vi "p6.2.vi"() -> ()   [LabVIEW 2020]
panel:
  in  "Kw":dbl=2.0
  in  "N FFT dBV":i32=4096
  out "FFT dBV":dbl[](graph)
  in  "N FFT":i32=1024
  out "FFT":dbl[](graph)=[1.1102230246251565e-16, 0.1179404859776075, 0.41931414977318965, 0.7678697584481545, 0.9999999999999988, 0.9969135645094994, 0.7439410887048731, 0.34832600660220614, 4.3813988651205395e-16, -0.11515526215938783, 0.08700222996580775, 0.5306405355054225, 0.9999999999999997, 1.2397845389517068, 1.0922522743307335, 0.5984660918442707, 5.761955295844675e-16, -0.3743504024510719, -0.28699300761890545, 0.26039872656253404, 0.9999999999999997, 1.5233277475171119, 1.5039874509749693, 0.8979000853754242, 9.418075112973702e-16, -0.6926899491581942, -0.7523921491322665, -0.08040357528638686, 0.9999999999999998, 1.8908459734075165, 2.0452675115378183, 1.297288147417813, 9.08683004564401e-16, -1.1302804118304979, -1.4022740708363133, -0.5640918868488319, 1.0000000000000009, 2.430632585174213, 2.8548321612466925, 1.9060608537435746, 8.633112624768329e-16, -1.8249724926294415, -2.4568882184753864, -1.3674473641410647, 0.9999999999999997, 3.373989764053941, 4.310015993746622, 3.033921208946577, 3.612083235008795e-16, -3.2028711087728787, -4.6315288740934175, -3.0963415349348566, 0.9999999999999983, 5.6186233099847, 7.986040899784292, 6.084571725761597, 1.1893112847244443e-17, -7.629629162693573, -12.443245049139438, -10.223584372481056, 0.9999999999999952, 19.621619548856494, 40.628968402289644, 57.33600236327664, 64.0, 58.189610616642796, 41.83638559111921, 20.475666946026298, 1.0000000000000062, -11.07851134787117, -13.653150976397987, -8.485878741428298, -6.022881901310196e-16, 6.942590842860555, 9.200953695486772, 6.478864158519104, 1.0000000000000013, -3.959262953429805, -5.854026322970516, -4.068940018683909, -6.904390630761646e-16, 3.903614113749591, 5.542767590086527, 4.2477943223758015, 1.0000000000000004, -2.245864050443687, -3.702690034497498, -2.7085163602699627, -5.049791833514398e-16, 2.795263416798454, 4.1166457149068005, 3.3260438372759777, 1.0000000000000013, -1.4662824774882115, -2.683270621160191, -2.039844003183214, -2.170775191704935e-16, 2.214843977835635, 3.3488795541278797, 2.8170416573555173, 1.0, -1.015918173819969, -2.0823743678223012, -1.638237350146765, -2.802329447010364e-16, 1.8542327387573896, 2.8644900582088124, 2.4912408081149704, 0.9999999999999998, -0.7199372125225274, -1.6826513579375895, -1.368004159637688, -1.9141313440356134e-16, 1.6063908514052578, 2.5282979870131013, 2.262998229774303, 1.0000000000000004, -0.5089521012657334, -1.3953985410182903, -1.172297267778555, -3.146002024872098e-16, 1.4242776832916586, 2.279579211474906, 2.0930359149462237, 1.0000000000000009, -0.3498973832944252, -1.177589687467472, -1.0230729827920086, -1.1102230246251565e-16, 1.2839457889263184, 2.086963203899523, 1.9607756213305376, 0.9999999999999979, -0.22498729289543584, -1.0057930871874996, -0.9048764059873323, -3.3156903224075413e-16, 1.1718985945518754, 1.9325817258102902, 1.854376125218883, 0.9999999999999993, -0.12378779585330946, -0.8661359730820365, -0.8084760751628219, -2.5961447105335884e-16, 1.079937445429123, 1.805493132107392, 1.7665299104018597, 0.9999999999999998, -0.03976364489568335, -0.7498675698744144, -0.7280087595690945, -1.8117081492085738e-16, 1.0027861665222886, 1.6986115457472104, 1.692475526467657, 1.0000000000000004, 0.03139373103987397, -0.6511860229171327, -0.659565671169491, 3.6300547937882384e-16, 0.9368899905228918, 1.6071386127083909, 1.6289726398344098, 1.0000000000000004, 0.09264459718003304, -0.5660866954941712, -0.6004366807305865, -6.324682132732809e-17, 0.8797627697518088, 1.5277043523073326, 1.573736161354584, 0.9999999999999997, 0.1460931335445112, -0.4917121383939054, -0.5486807565835418, 4.0980327146294453e-17, 0.829610923760691, 1.4578690017292486, 1.5251060530083156, 0.9999999999999989, 0.1932781902090958, -0.4259658383974144, -0.502869236821099, -4.6054350386270707e-17, 0.7851061629724353, 1.39582030989787, 1.4818456190947975, 1.0, 0.23535273620404806, -0.3672726425755104, -0.46192581425597223, -4.373283541979666e-15, 0.7452424853713986, 1.3401821981695914, 1.4430134324972246, 1.0000000000000016, 0.27319879874284864, -0.3144246548035006, -0.4250231798408728, -5.765073530784608e-17, 0.7092430573891835, 1.2898896749431539, 1.407879283999169, 1.0000000000000004, 0.3075034639506445, -0.26647896463208864, -0.3915141824632936, -2.569405885103387e-16, 0.6764977556871281, 1.2441046492473682, 1.375867423065904, 1.0000000000000002, 0.33881053754760826, -0.22268790693642482, -0.3608847377843961, -1.1216207552939258e-16, 0.6465201785095566, 1.2021578130944914, 1.346517258633479, 0.9999999999999998, 0.367556520694475, -0.18245035866530035, -0.3327208507493926, -2.0915206164717483e-16, 0.6189173774805913, 1.1635076123796106, 1.319455542642623, 0.9999999999999992, 0.39409620457404093, -0.14527700279036404, -0.306685037421258, -1.483504445482778e-16, 0.5933681118883954, 1.1277107004929205, 1.2943762918084158, 0.9999999999999997, 0.41872122928599304, -0.11076508451318334, -0.2824991521781703, 2.1456919189062408e-16, 0.5696069419679941, 1.0944002797150552, 1.2710260387533467, 1.0, 0.44167377261346097, -0.07857975438129544, -0.25993167065099493, -5.4812654630920924e-17, 0.5474124035024525, 1.0632699689796672, 1.2491928257074043, 1.0000000000000009, 0.46315680309159735, -0.04844006863312339, -0.23878813002643842, 1.1102230246251565e-16, 0.5265980870349921, 1.0340616130406408, 1.228697873020515, 0.999999999999999, 0.4833418674319925, -0.02010833860070249, -0.2189038443902526, 1.0774697208352187e-17, 0.5070058182427253, 1.0065559483160782, 1.2093891900458458, 1.0000000000000004, 0.5023750807405464, 0.006618074258630147, -0.20013828443372872, -9.426726095832825e-18, 0.4885003809837876, 0.9805653698008545, 1.191136617114367, 1.0000000000000004, 0.5203817880562114, 0.03191315222460833, -0.18237069175541068, -1.250443610060071e-16, 0.4709653884274459, 0.9559282641509659, 1.1738279359708557, 1.000000000000001, 0.5374702307723851, 0.055927256648473644, -0.16549662066033533, 3.661613075155523e-16, 0.45430001928672326, 0.9325045246566586, 1.1573657876909524, 0.9999999999999996, 0.5537344588335508, 0.07879113216086642, -0.14942518492306, -1.9455002627372058e-16, 0.4384164134139906, 0.9101719682559929, 1.14166520771626, 0.9999999999999999, 0.5692566649792242, 0.10061911970433401, -0.13407684616647514, 3.4191338006119983e-16, 0.42323757527524464, 0.8888234482272754, 1.126651637422651, 0.999999999999999, 0.584109071598281, 0.12151175637872436, -0.11938162251528944, 5.576196745660244e-17, 0.40869567245468286, 0.8683645086157401, 1.1122593072005698, 1.0000000000000002, 0.5983554679957568, 0.1415578956068123, -0.1052776263855002, -2.7321438156213356e-15, 0.39473064420570336, 0.8487114643106126, 1.0984299117525964, 1.0000000000000009, 0.6120524721044411, 0.16083644880718717, -0.09170986224846123, 2.7867324893886046e-16, 0.3812890553987795, 0.8297898183572044, 1.085111517140453, 1.000000000000002, 0.6252505732304984, 0.17941782601104883, -0.07862923137992439, -1.2595311869715562e-16, 0.36832314621916484, 0.8115329485291602, 1.0722576530408452, 1.0000000000000009, 0.6379949994857299, 0.1973651352229009, -0.06599170262845944, 1.2064589217501586e-16, 0.35579003915045104, 0.7938810104409895, 1.059826554075753, 0.9999999999999999, 0.6503264438692102, 0.21473518709895312, -0.05375761726538386, -5.200147252472014e-16, 0.34365107319520566, 0.7767800159741998, 1.047780521932358, 0.9999999999999992, 0.6622816756358763, 0.23157934150755133, -0.041891102818139625, -9.209173112415381e-17, 0.33187124167413207, 0.7601810545266237, 1.0360853859605232, 0.9999999999999993, 0.6738940580038386, 0.24794422489511148, -0.03035957601554584, 5.447200525856749e-17, 0.3204187148378739, 0.7440396312907017, 1.0247100445183381, 0.9999999999999993, 0.6851939889579275, 0.26387234150129735, -0.019133318999220328, 1.5619315264521672e-17, 0.3092644323016204, 0.7283151019390508, 1.0136260728795885, 0.9999999999999994, 0.696209278580651, 0.27940259690841895, -0.008185116079658439, -1.1102230246251565e-16, 0.2983817532482379, 0.7129701871205936, 1.0028073862765414, 1.0, 0.7069654737464687, 0.2945707488502367, 0.002510059242883722, 1.9499375925659952e-16, 0.2877461546437976, 0.6979705533240912, 0.9922299488153357, 1.0000000000000009, 0.7174861389770005, 0.3094097974072807, 0.012975315351816397, -1.3729331391229953e-17, 0.2773349695200261, 0.6832844491524461, 0.9818715207088378, 1.0000000000000002, 0.727793100643996, 0.3239503245028259, 0.023232078520840305, 1.8424880760427233e-16, 0.2671271588133646, 0.6688823880234691, 0.9717114376270775, 1.0, 0.7379066604263154, 0.3382207908533479, 0.03330029948260793, 6.0068273302116e-17, 0.25710311139426656, 0.6547368698858937, 0.961730417047242, 0.9999999999999983, 0.7478457829040923, 0.35224779711982146, 0.043198635220118575, 2.0085736670586172e-16, 0.24724446783664233, 0.6408221358002484, 0.9519103873526054, 0.9999999999999996, 0.7576282613516778, 0.3660563148755007, 0.05294460986335392, 6.054662715253032e-16, 0.23753396421470674, 0.6271139502492646, 0.9422343361285794, 0.9999999999999996, 0.7672708651285118, 0.3796698920936077, 0.06255475794556453, 2.830317846248932e-16, 0.2279552928101376, 0.6135894068629515, 0.9326861746691026, 0.9999999999999991, 0.7767894715311563, 0.3931108371200729, 0.07204475276506273, 0.0, 0.21849297709504611, 0.6002267539083235, 0.9232506161646139, 1.0000000000000004, 0.7861991845348033, 0.4064003844972186, 0.08142952218557653, 7.663316195753589e-17, 0.2091322587483071, 0.587005236433999, 0.9139130654150138, 1.0000000000000009, 0.7955144424991474, 0.4195588455172756, 0.09072335387249297, -2.7623553195001815e-16, 0.19985899478133828, 0.5739049523989566, 0.9046595182137667, 1.0, 0.804749116626427, 0.43260574598880264, 0.099939991689877, -3.0987641487582927e-16, 0.1906595631083664, 0.5609067204713905, 0.8954764687946128, 0.9999999999999991, 0.8139166017260543, 0.44555995337800164, 0.10909272476172771, -7.516737586960234e-16, 0.1815207751058886, 0.5479919574723923, 0.8863508239315387, 0.9999999999999993, 0.8230299006521319, 0.45843979522759404, 0.11819447052275545, -2.991660226013099e-16, 0.17242979387485868, 0.535142563671349, 0.8772698224420669, 0.9999999999999997, 0.8321017036291152, 0.47126317054859534, 0.12725785294137026, -3.710530637896763e-16, 0.163374057053591, 0.5223408143246283, 0.8682209589707324, 0.9999999999999999, 0.8411444635616836, 0.48404765571679864, 0.13629527698555605, 4.145423111735749e-17, 0.15434120313442523, 0.5095692559928563, 0.8591919110279486, 0.9999999999999997, 0.8501704683330381, 0.4968106062803564, 0.1453190003167287, 1.1102230246251565e-16]
  out "error out":errorcluster
  in  "stop":bool
  in  "fs DA (Hz)":dbl=8000.0
  in  "fs AD (Hz)":dbl=8000.0
  in  "device name":tag="myDAQ1"
  in  "L":i32=128
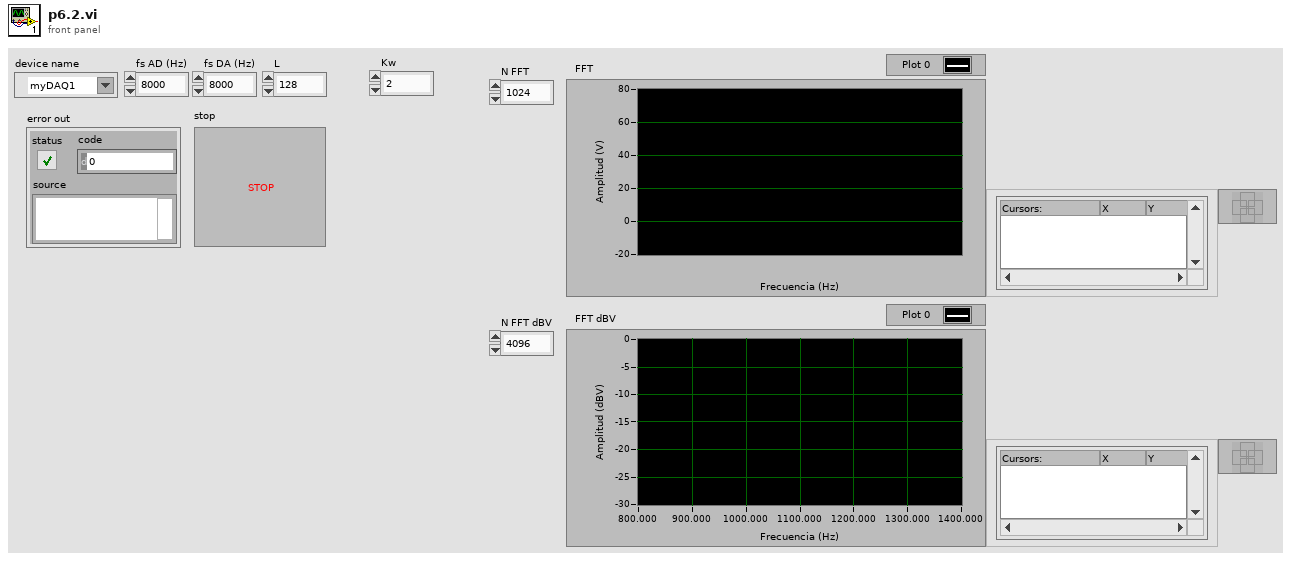
[diagram p1: front panel]
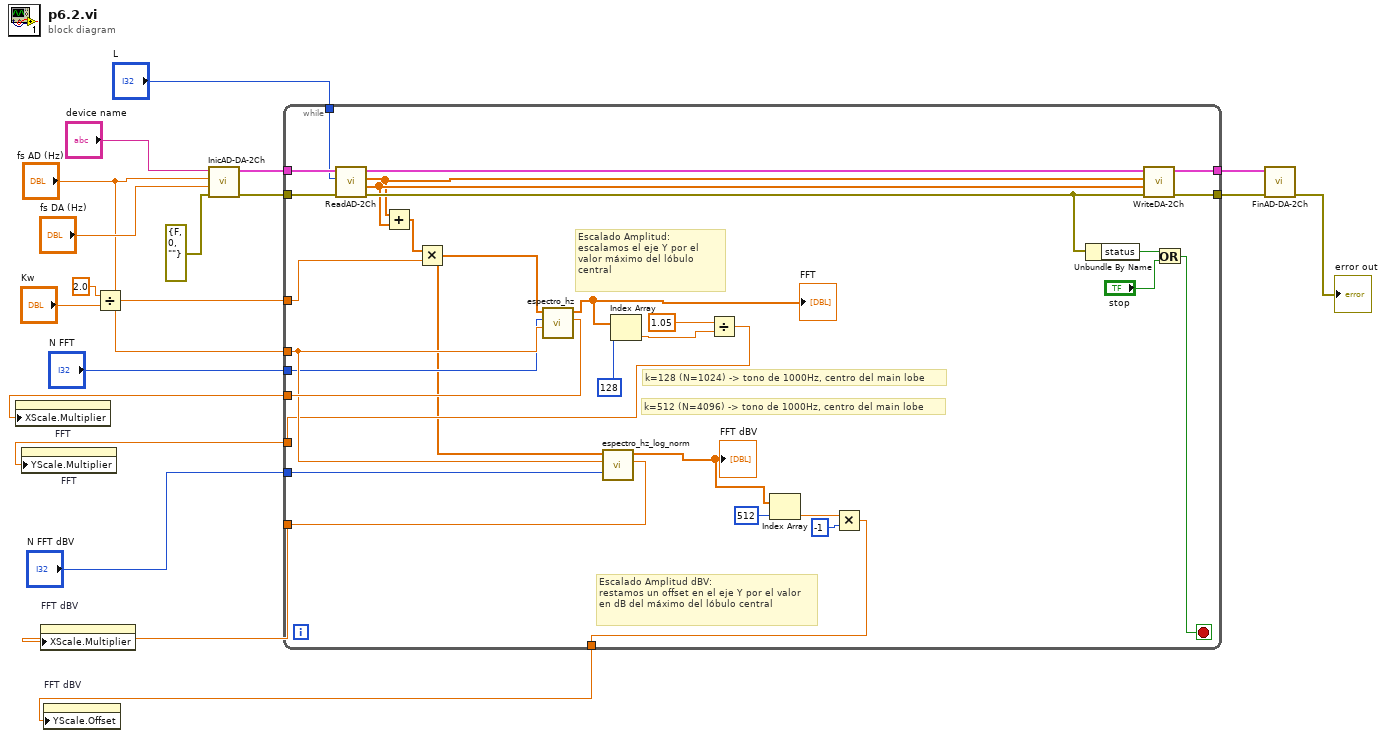
[diagram p0: block diagram]
diagram:
  n1 = Divide(x=2.0, y="Kw") -> (x/y=w9:dbl)
  n2 = call <userlib>:"InicAD-DA-2Ch.vi"("error in"=errorcluster {"status"=FALSE, "code"=0, "source"=""}, "fs DA (Hz)"="fs DA (Hz)", "fs AD (Hz)"="fs AD (Hz)", "device name"="device name") -> ("error out"=w16:errorcluster, "Tarea Out"=w17:cluster{"AD":refnum<k21>, "DA":refnum<k21>})  [unwired: 6 in]
  n3 = while {
    tunnel: [w49] -> w19
    tunnel: [w48] -> w18
    tunnel: w17 -> [w47]
    tunnel: w16 -> [w46]
    tunnel: "fs AD (Hz)" -> [w38]
    tunnel: w9 -> [w40]
    tunnel: "N FFT" -> [w33]
    tunnel: [w39] -> w7
    tunnel: [w32] -> w3
    tunnel: "N FFT dBV" -> [w34]
    tunnel: [w29] -> w4
    tunnel: [w26] -> w2
    tunnel: "L" -> [w24]
    stop <- w41 stop-if-true
    # "k=512 (N=4096) -> tono de 1000Hz, centro del main lobe"
    # "Escalado Amplitud dBV:\nrestamos un offset en el eje Y por el valor en dB del máximo del lóbulo central"
    # "k=128 (N=1024) -> tono de 1000Hz, centro del main lobe"
    # "Escalado Amplitud:\nescalamos el eje Y por el valor máximo del lóbulo central"
    n4 = call <userlib>:"ReadAD-2Ch.vi"("error in"=w46, "numero de muestras"=w24, "Tarea In"=w47) -> ("error out"=w44:errorcluster, "Data Right"=w23:dbl[], "Data Left"=w21:dbl[], "Tarea Out"=w45:cluster{"AD":refnum<k21>, "DA":refnum<k21>})  [unwired: 5 in]
    n5 = Add(x=w21, y=w23) -> (x+y=w22:dbl[])
    n6 = Multiply(x=w22, y=w40) -> (x*y=w20:dbl[])
    n7 = call "espectro_hz.vi"("fs"=w38, "N FFT"=w33, "X"=w20) -> ("XScale"=w39:dbl, "FFT(X)"=w31:cdb[])  [unwired: 7 in]
    "FFT" <- w31
    n8 = call "espectro_hz_log_norm.vi"("N FFT dBV"=w34, "fs AD (Hz)"=w38, "Array in"=w20) -> ("XScale"=w32:dbl, "Array out"=w25:cdb[])  [unwired: 7 in]
    "FFT dBV" <- w25
    n9 = Index Array(array=w31, index=128) -> (element=w37:cdb)
    n10 = Divide(x=1.05, y=w37) -> (x/y=w29:cdb)
    n11 = Index Array(array=w25, index=512) -> (element=w28:cdb)
    n12 = Multiply(x=w28, y=-1 ("index")) -> (x*y=w26:cdb)
    n13 = Unbundle By Name(w44) -> ("status"=w43:bool)
    n14 = call <userlib>:"WriteDA-2Ch.vi"("error in"=w44, "Data Right"=w23, "Data Left"=w21, "Tarea In"=w45) -> ("error out"=w48:errorcluster, "Tarea Out"=w49:cluster{"AD":refnum<k21>, "DA":refnum<k21>})  [unwired: 6 in]
    n15 = Or(x=w43, y="stop") -> (x .or. y?=w41:bool)
  }
  n16 = property on="FFT" class="WFGraph (strict)"("XScale.Multiplier"=w7) -> ()  [unwired: 2 in, 2 out]
  n17 = property on="FFT" class="WFGraph (strict)"("YScale.Multiplier"=w4) -> ()  [unwired: 2 in, 2 out]
  n18 = property on="FFT dBV" class="WFGraph (strict)"("XScale.Multiplier"=w3) -> ()  [unwired: 2 in, 2 out]
  n19 = property on="FFT dBV" class="WFGraph (strict)"("YScale.Offset"=w2) -> ()  [unwired: 2 in, 2 out]
  n20 = call <userlib>:"FinAD-DA-2Ch.vi"("error in"=w18, "Tarea In"=w19) -> ("error out"=→"error out":errorcluster)  [unwired: 9 in]
